vi "Make Receiver.vi"(8 "error in (no error)":errorcluster, 11 "Concrete Message Scripter in":refnum<class "Concrete Message Scripter.lvclass">) -> (0 "error out":errorcluster, 3 "Concrete Message Scripter out":refnum<class "Concrete Message Scripter.lvclass">)   [LabVIEW 2020, in "Message Maker.lvlib" / "Concrete Message Scripter.lvclass"]
uses:
  Concrete Message Scripter.lvclass
  Concrete Message Scripter.lvclass/Concrete Message Scripter.ctl
  Message Scripter/Message Scripter.lvclass
  Message Maker.lvlib
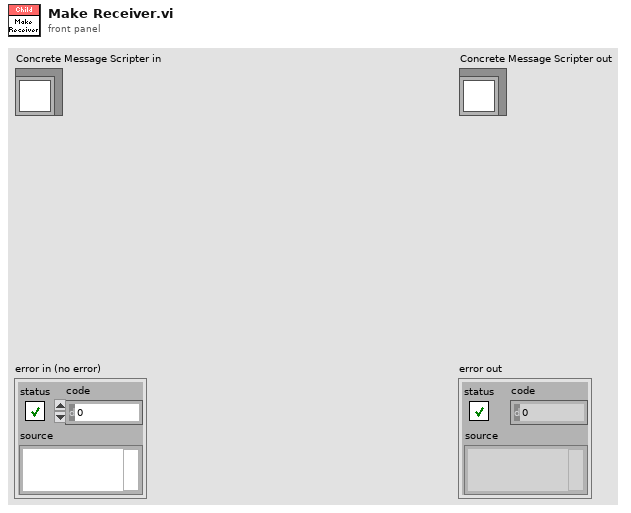
[diagram p1: front panel]
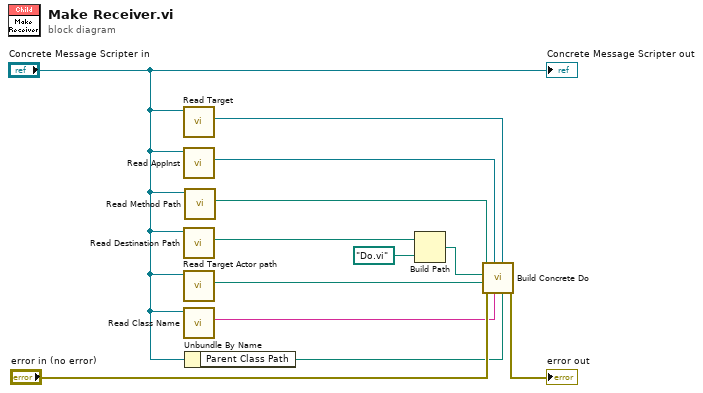
[diagram p0: block diagram]
diagram:
  n1 = call "Read Target.vi"("Message Scripter in"="Concrete Message Scripter in") -> ("Target"=w1:refnum<vi>)  [unwired: 10 in]
  n2 = call "Read AppInst.vi"("Message Maker in"="Concrete Message Scripter in") -> ("AppInst"=w11:refnum<vi>)  [unwired: 10 in]
  n3 = call "Read Destination Path.vi"("Message Scripter in"="Concrete Message Scripter in") -> ("Destination Path"=w10:path)  [unwired: 10 in]
  n4 = call "Read Target Actor path.vi"("Message Scripter in"="Concrete Message Scripter in") -> ("Target Actor path"=w12:path)  [unwired: 10 in]
  n5 = call "Read Class Name.vi"("Message Scripter in"="Concrete Message Scripter in") -> ("Class Name"=w4:string)  [unwired: 10 in]
  n6 = call "Read Method Path.vi"("Message Maker in"="Concrete Message Scripter in") -> ("Method Path"=w3:path)  [unwired: 10 in]
  n7 = Unbundle By Name("Concrete Message Scripter in") -> ("Parent Class Path"=w5:path)
  n8 = Build Path(base path=w10, name or relative path=path "Do.vi") -> (appended path=w8:path)
  n9 = call "Build Concrete Do.vi"("Abstract class path"=w5, "Target"=w1, "Class Name"=w4, "AppInst"=w11, "error in (no error)"="error in (no error)", "Actor class path"=w12, "Do Method path"=w8, "Target Actor Method path"=w3) -> ("error out"=→"error out":errorcluster)  [unwired: 3 in]
  "Concrete Message Scripter out" <- "Concrete Message Scripter in"
